vi "save_data (SubVI).vi"(6 "Process list":T1, 7 "environ cluster":cluster{dbl[], dbl[]}, 8 "DC volts arr":dbl[](array[numeric]), 9 "Sample rate":dbl format="%#_13g", 10 "Filename":path, 11 "data":i16[][](array[numeric])) -> ()   [LabVIEW 2014]
uses:
  <vilib>/addons/h5labview2/file/H5Fmode.ctl
  <vilib>/addons/h5labview2/base/lib_path.vi
  <vilib>/addons/h5labview2/base/H5Equery.vi
  <vilib>/addons/h5labview2/dataset/H5Dwrite.llb/H5Dwrite.xnode
  <vilib>/addons/h5labview2/attrib/H5Awrite.llb/H5Awrite.xnode
  <vilib>/addons/h5labview2/base/hid_t.ctl
  <vilib>/addons/h5labview2/file/H5F.lvlib
  <vilib>/addons/h5labview2/group/H5G.lvlib
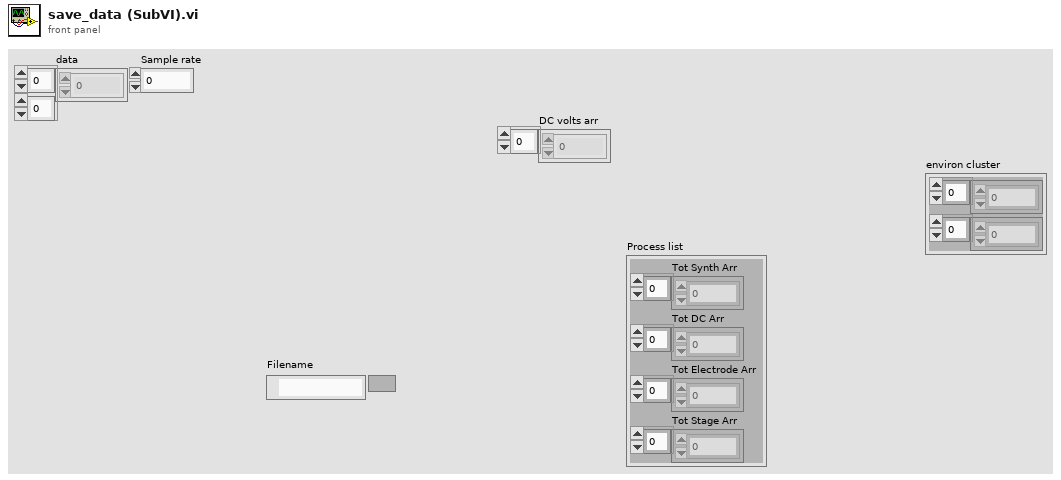
[diagram p1: front panel]
types:
  T1 = cluster{"Tot Synth Arr":dbl[], "Tot DC Arr":dbl[], "Tot Electrode Arr":dbl[], "Tot Stage Arr":dbl[]}
  T2 = typedef "H5F.lvlib/H5Fmode.ctl" = enum16{"read-only", "read-write", "overwrite", "create new", "open or create"}
  T3 = typedef "hid_t.ctl" = i32
  T4 = cluster{"Sample rate":dbl, dbl, dbl[], dbl[], "Tot Synth Arr":dbl[], "Tot DC Arr":dbl[], "Tot Electrode Arr":dbl[], "DC volts arr":dbl[], "Tot Stage Arr":dbl[]}
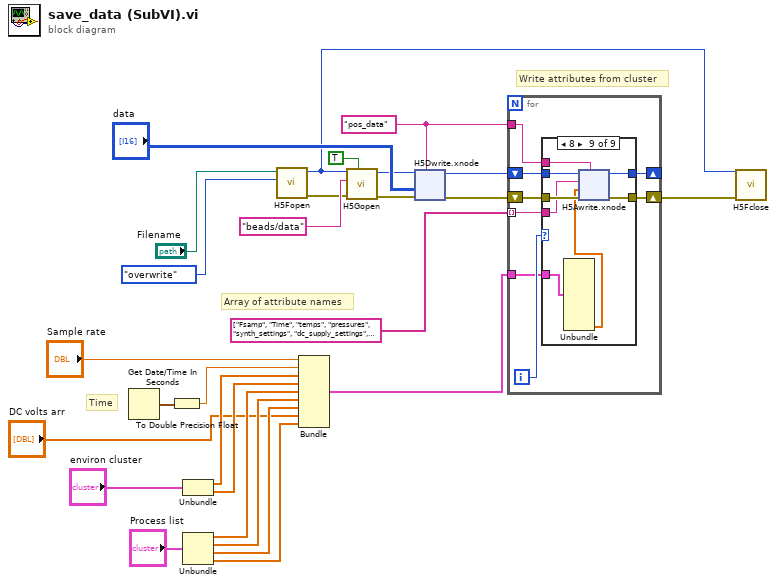
[diagram p0: block diagram]
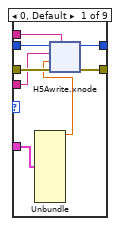
[diagram p2: hidden frame]
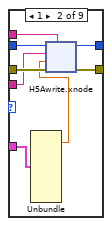
[diagram p3: hidden frame]
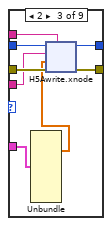
[diagram p4: hidden frame]
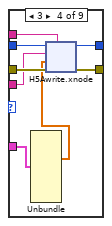
[diagram p5: hidden frame]
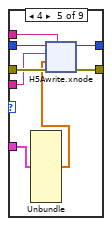
[diagram p6: hidden frame]
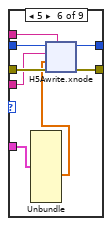
[diagram p7: hidden frame]
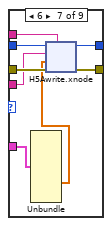
[diagram p8: hidden frame]
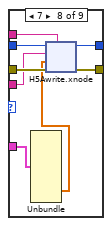
[diagram p9: hidden frame]
diagram:
  w27 = "pos_data" ("dataset name")
  # "Time"
  # "Array of attribute names"
  # "Write attributes from cluster"
  n1 = Get Date/Time In Seconds() -> (seconds since 1Jan1904=w22:timestamp)
  n2 = To Double Precision Float(number=w22) -> (double precision float=w12:dbl)
  n3 = Unbundle("environ cluster") -> (w11:dbl[], w10:dbl[])
  n4 = Unbundle("Process list") -> ("Tot Synth Arr"=w5:dbl[], "Tot DC Arr"=w4:dbl[], "Tot Electrode Arr"=w3:dbl[], "Tot Stage Arr"=w2:dbl[])
  n5 = call <vilib>:"H5Fopen.vi"("mode (read-only)"=H5Fmode."overwrite", "path"="Filename") -> ("error out"=w18:errorcluster, "ref out"=w7:T3)  [unwired: 8 in]
  n6 = Bundle("Sample rate"="Sample rate", w12, w11, w10, "Tot Synth Arr"=w5, "Tot DC Arr"=w4, "Tot Electrode Arr"=w3, "DC volts arr"="DC volts arr", "Tot Stage Arr"=w2) -> (w9:T4)  [unwired: 1 in]
  n7 = call <vilib>:"H5Gopen.vi"("create? (F)"=TRUE, "error in (no error)"=w18, "name"="beads/data", "ref in"=w7) -> ("error out"=w24:errorcluster, "group out"=w8:T3)  [unwired: 6 in]
  n8 = xnode "H5Dwrite.xnode"("dataset name"=w27, "error in (no error)"=w24, "data"="data", "ref in"=w8) -> ("error out"=w23:errorcluster, "ref out"=w16:i32)  [unwired: 3 in, 1 out]
  n9 = for {
    tunnel: w27 -> [w35]
    shift-right: [w33] -> _
    shift-left: w16 -> [w30]
    shift-right: [w32] -> w20
    shift-left: w23 -> [w34]
    tunnel: string[] ["Fsamp", "Time", "temps", "pressures", "synth_settings", "dc_supply_settings", "electrode_settings", "electrode_dc_vals", "stage_settings"] -> [w31] mode=indexing
    tunnel: w9 -> [w28]
    i -> [w29]
    n10 = case shown="8" w29 {
      tunnel: w35 -> [w43 w69 w95 w121 w147 w173 w199 w225 w251]
      tunnel: w34 -> [w42 w68 w94 w120 w146 w172 w198 w224 w250]
      tunnel: [w41 w67 w93 w119 w145 w171 w197 w223 w249] -> w33
      tunnel: [w40 w66 w92 w118 w144 w170 w196 w222 w248] -> w32
      tunnel: w31 -> [w39 w65 w91 w117 w143 w169 w195 w221 w247]
      tunnel: w30 -> [w38 w64 w90 w116 w142 w168 w194 w220 w246]
      tunnel: w28 -> [w37 w63 w89 w115 w141 w167 w193 w219 w245]
      frame 0, Default {
        n11 = Unbundle(w37) -> ("Sample rate"=w36:dbl)  [unwired: 8 out]
        n12 = xnode "H5Awrite.xnode"("object name"=w43, "error in (no error)"=w42, "data"=w36, "attrib name"=w39, "ref in"=w38) -> ("error out"=w40:errorcluster, "ref out"=w41:T3)  [unwired: 2 in, 1 out]
      }
      frame 1 {
        n13 = Unbundle(w63) -> (w62:dbl)  [unwired: 8 out]
        n14 = xnode "H5Awrite.xnode"("object name"=w69, "error in (no error)"=w68, "data"=w62, "attrib name"=w65, "ref in"=w64) -> ("error out"=w66:errorcluster, "ref out"=w67:T3)  [unwired: 2 in, 1 out]
      }
      frame 2 {
        n15 = Unbundle(w89) -> (w88:dbl[])  [unwired: 8 out]
        n16 = xnode "H5Awrite.xnode"("object name"=w95, "error in (no error)"=w94, "data"=w88, "attrib name"=w91, "ref in"=w90) -> ("error out"=w92:errorcluster, "ref out"=w93:T3)  [unwired: 2 in, 1 out]
      }
      frame 3 {
        n17 = Unbundle(w115) -> (w114:dbl[])  [unwired: 8 out]
        n18 = xnode "H5Awrite.xnode"("object name"=w121, "error in (no error)"=w120, "data"=w114, "attrib name"=w117, "ref in"=w116) -> ("error out"=w118:errorcluster, "ref out"=w119:T3)  [unwired: 2 in, 1 out]
      }
      frame 4 {
        n19 = Unbundle(w141) -> ("Tot Synth Arr"=w140:dbl[])  [unwired: 8 out]
        n20 = xnode "H5Awrite.xnode"("object name"=w147, "error in (no error)"=w146, "data"=w140, "attrib name"=w143, "ref in"=w142) -> ("error out"=w144:errorcluster, "ref out"=w145:T3)  [unwired: 2 in, 1 out]
      }
      frame 5 {
        n21 = Unbundle(w167) -> ("Tot DC Arr"=w166:dbl[])  [unwired: 8 out]
        n22 = xnode "H5Awrite.xnode"("object name"=w173, "error in (no error)"=w172, "data"=w166, "attrib name"=w169, "ref in"=w168) -> ("error out"=w170:errorcluster, "ref out"=w171:T3)  [unwired: 2 in, 1 out]
      }
      frame 6 {
        n23 = Unbundle(w193) -> ("Tot Electrode Arr"=w192:dbl[])  [unwired: 8 out]
        n24 = xnode "H5Awrite.xnode"("object name"=w199, "error in (no error)"=w198, "data"=w192, "attrib name"=w195, "ref in"=w194) -> ("error out"=w196:errorcluster, "ref out"=w197:T3)  [unwired: 2 in, 1 out]
      }
      frame 7 {
        n25 = Unbundle(w219) -> ("DC volts arr"=w218:dbl[])  [unwired: 8 out]
        n26 = xnode "H5Awrite.xnode"("object name"=w225, "error in (no error)"=w224, "data"=w218, "attrib name"=w221, "ref in"=w220) -> ("error out"=w222:errorcluster, "ref out"=w223:T3)  [unwired: 2 in, 1 out]
      }
      frame 8 {
        n27 = Unbundle(w245) -> ("Tot Stage Arr"=w244:dbl[])  [unwired: 8 out]
        n28 = xnode "H5Awrite.xnode"("object name"=w251, "error in (no error)"=w250, "data"=w244, "attrib name"=w247, "ref in"=w246) -> ("error out"=w248:errorcluster, "ref out"=w249:T3)  [unwired: 2 in, 1 out]
      }
    }
  }
  n29 = call <vilib>:"H5Fclose.vi"("error in (no error)"=w20, "ref"=w7) -> ()  [unwired: 9 in, 1 out]
